vi "Get Mouse Position.vi"(8 "error in (no error)":errorcluster) -> (0 "error out":errorcluster, 3 "Mouse Position":cluster{"Horizontal":i32, "Vertical":i32})   [LabVIEW 2021, in "Panel Movement Center Maximize.lvlib"]
doc: "This VI will return the <B>Mouse Position</B> relative to the upper left corner of the screen. This VI will get the position regardless of what window has focus.\n\n-----\nHooovahh\n(Brian Hoover)"
uses:
  <vilib>/Utility/inputDevices.llb/mouseAcquire.vi
  <vilib>/Utility/inputDevices.llb/closeMouse.vi
  Panel Movement Center Maximize.lvlib
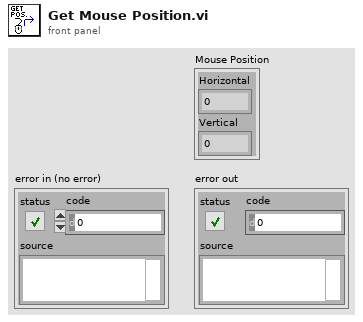
[diagram p1: front panel]
types:
  T1 = cluster{"Horizontal":i32, "Vertical":i32, "Scrolling":i32}
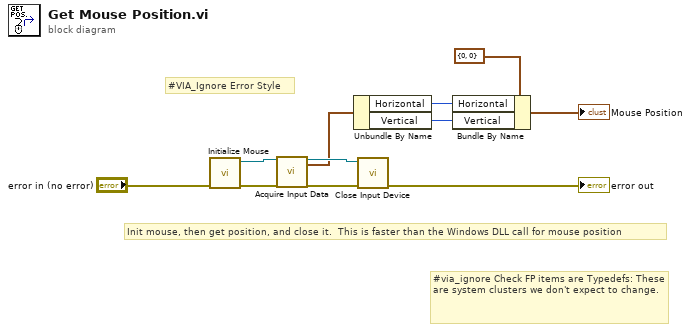
[diagram p0: block diagram]
diagram:
  # "#via_ignore Check FP items are Typedefs: These are system clusters we don't expect to change."
  # "#VIA_Ignore Error Style"
  # "Init mouse, then get position, and close it.  This is faster than the Windows DLL call for mouse position"
  n1 = call <vilib>:"Initialize Mouse.vi"("error in (no error)"="error in (no error)") -> ("error out"=w5:errorcluster, "device ID"=w8:refnum<k1>)  [unwired: 9 in]
  n2 = call-poly <vilib>:"Acquire Input Data.vi"("device ID"=w8, "error in (no error)"=w5) -> ("device ID"=w7:refnum<k1>, "axis info"=w4:T1, "error out"=w6:errorcluster)  [unwired: 14 in, 1 out]
  n3 = Unbundle By Name(w4) -> ("Horizontal"=w2:i32, "Vertical"=w1:i32)
  n4 = call-poly <vilib>:"Close Input Device.vi"("error in (no error)"=w6, "device ID"=w7) -> ("error out"=→"error out":errorcluster)  [unwired: 8 in]
  n5 = Bundle By Name(cluster=cluster{"Horizontal":i32, "Vertical":i32} {"Horizontal"=0, "Vertical"=0} ("Mouse Position"), "Horizontal"=w2, "Vertical"=w1) -> (→"Mouse Position":cluster{"Horizontal":i32, "Vertical":i32})
